vi "W2E.vi"() -> ()   [LabVIEW 2021]
panel:
  in  "stop":bool
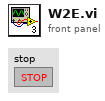
[diagram p1: front panel]
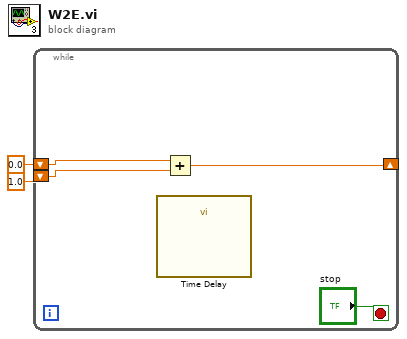
[diagram p0: block diagram]
diagram:
  n1 = while {
    shift-right: [w4] -> _
    shift-left: 0.0 -> [w6]
    shift-left: 1.0 -> [w5]
    stop <- "stop" stop-if-true
    n2 = call "Time Delay"() -> ()  [unwired: 11 in, 1 out]
    n3 = Add(x=w6, y=w5) -> (x+y=w4:dbl)
  }
